vi "Storage Tele-Op.vi"(8 "Operator Buttons":bool[](array[boolean]), 9 "Operator Axes":dbl[](array[numeric]), 10 "Driver Buttons":bool[](array[boolean]), 11 "Driver Axes":dbl[](array[numeric])) -> ()   [LabVIEW 2019]
uses:
  Implementation/Storage Operations.ctl
  15c8f0b7-f024-43b2-a055-fc2d36092548.vi
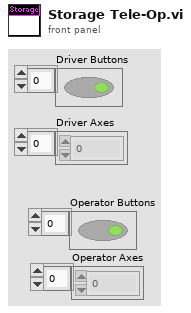
[diagram p1: front panel]
types:
  T1 = typedef "Storage Operations.ctl" = enum16{"Reserve", "Read Current", "Immediate", "Intake", "Shoot", "Override"}
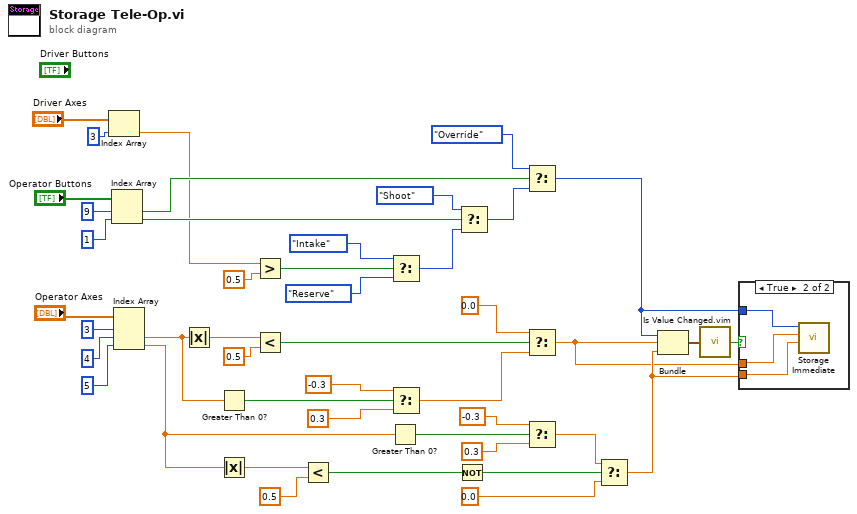
[diagram p0: block diagram]
diagram:
  n1 = Index Array(array="Driver Axes", index=3) -> (element=w5:dbl)
  n2 = Index Array(array="Operator Buttons", index #1=9 ("B"), index #2=1 ("index")) -> (element #1=w14:bool, element #2=w13:bool)
  n3 = Index Array(array="Operator Axes", index #1=3 ("index"), index #2=4 ("index"), index #3=5 ("index")) -> (element #2=w30:dbl, element #3=w29:dbl)  [unwired: 1 out]
  n4 = Absolute Value(x=w30) -> (abs(x)=w33:dbl)
  n5 = Greater Than 0?(x=w30) -> (x > 0?=w27:bool)
  n6 = Absolute Value(x=w29) -> (abs(x)=w34:dbl)
  n7 = Greater?(x=w5, y=0.5) -> (0:w1:bool)
  n8 = Less?(x=w33, y=0.5) -> (x < y?=w22:bool)
  n9 = Less?(x=w34, y=0.5) -> (x < y?=w10:bool)
  n10 = Greater Than 0?(x=w29) -> (x > 0?=w28:bool)
  n11 = Select(t=Storage_Operations."Intake" ("Operation"), s=w1, f=Storage_Operations."Reserve" ("Operation")) -> (s? t:f=w42:T1)
  n12 = Select(t=-0.3, s=w27, f=0.3) -> (s? t:f=w26:dbl)
  n13 = Not(x=w10) -> (.not. x?=w11:bool)
  n14 = Select(t=Storage_Operations."Shoot" ("Operation"), s=w13, f=w42) -> (s? t:f=w38:T1)
  n15 = Select(t=Storage_Operations."Override", s=w14, f=w38) -> (s? t:f=w12:T1)
  n16 = Select(t=0.0, s=w22, f=w26) -> (s? t:f=w8:dbl)
  n17 = Select(t=-0.3, s=w28, f=0.3) -> (s? t:f=w25:dbl)
  n18 = Select(t=w25, s=w11, f=0.0 ("t")) -> (s? t:f=w9:dbl)
  n19 = Bundle("Operation"=w12, "f"=w8, "t"=w9) -> (w16:cluster{"Operation":T1, "f":dbl, "t":dbl})  [unwired: 1 in]
  n20 = call "Is Value Changed.vim"("value"=w16) -> ("changed or first call?"=w15:bool)
  n21 = case shown="True" w15 {
    tunnel: w12 -> [_ w47]
    tunnel: w9 -> [_ w45]
    tunnel: w8 -> [_ w46]
    frame False {
    }
    frame True {
      n22 = call "Storage Immediate.vi"("Transfer Speed"=w45, "Spindexer Speed"=w46, "Operation"=w47) -> ()  [unwired: 9 in]
    }
  }
